vi "York DIHB - Data Processing - SNR and FFT.vi"() -> ()   [LabVIEW 2020]
doc: "Load a raw data file and calculate signal to noise ratio (SNR) & fast fourier transform (FFT). \n\nDisplays the first/largest wave in the signal."
uses:
  <vilib>/Analysis/5stat.llb/RMS (DBL).vi
  <vilib>/Utility/file.llb/Read Delimited Spreadsheet (DBL).vi
  <vilib>/measure/mascope.llb/Amplitude and Levels 1 chan.vi
  <vilib>/measure/madcrms.llb/Basic Averaged DC-RMS for 1 Chan.vi
  <vilib>/measure/maspectr.llb/FFT Spectrum (Mag-Phase) for 1 Chan.vi
  <vilib>/measure/NI_MAPro.lvlib
  <vilib>/Analysis/NI_AALPro.lvlib
panel:
  out "Signal to Noise Ratio":dbl format="%#_3g"
  out "Signal RMS Voltage":dbl format="%0.4f"
  out "Noise RMS Voltage":dbl format="%0.4f"
  out "Samples":i32
  out "Noise FFT > 250 Hz":cluster{"f0":dbl, "df":dbl, "magnitude":dbl[]}(graph)
  out "Pulse FFT":cluster{"f0":dbl, "df":dbl, "magnitude":dbl[]}(graph)
  out "Noise FFT <250 Hz":cluster{"f0":dbl, "df":dbl, "magnitude":dbl[]}(graph)
  out "Noise - Peak to Peak (V)":dbl format="%.2p"
  out "Signal - First Pulse (Volts)":waveform(dbl)(graph)
  out "Detected Frequency (Hz)":dbl format="%.2p"
  out "Noise (Volts)":waveform(dbl)(graph)
  out "Pulse Start Time (ms)":dbl
  out "DC offset (V)":dbl format="%0.2p"
  out "Peak to Peak - Amplitude (V)":dbl format="%.2p"
  out "Maximum Signal (V)":dbl format="%.2g"
  out "Minimum Signal (V)":dbl format="%.2g"
  out "Samples":i32
  out "Sampling Rate (MHz)":dbl
  out "Sampling Period (s)":dbl
  out "Raw Data - Strain Amplifier Output (Volts)":waveform(dbl)(graph)
  out "Projectile Velocity (m/s)":dbl
  out "Strain Amplifier (Volts)":dbl[](array[numeric])
  out "Time (Seconds)":dbl[](array[numeric])
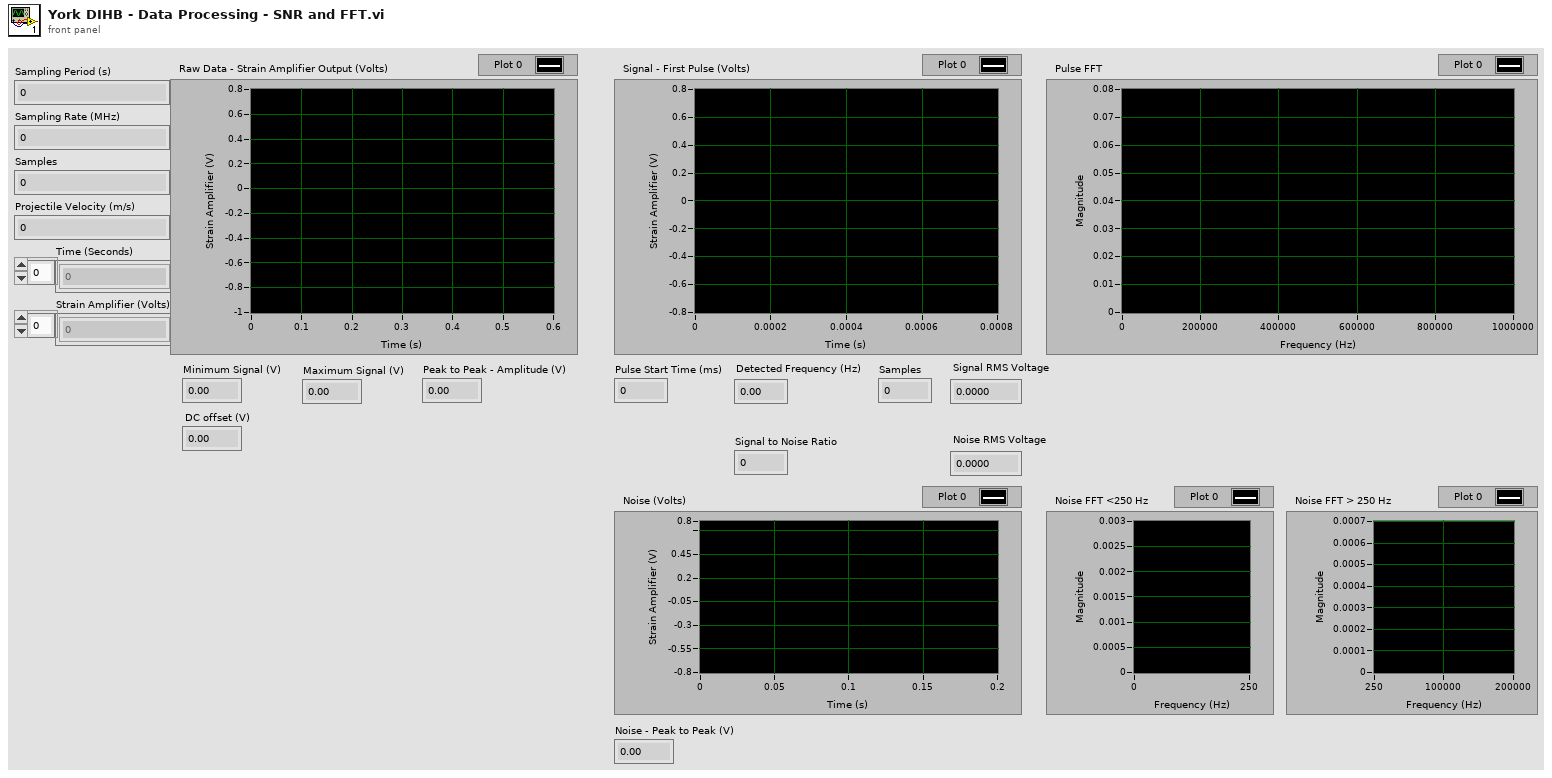
[diagram p1: front panel]
types:
  T1 = cluster{"method":enum32{"histogram", "peak", "auto select"}, "histogram size":i32, "histogram method":enum16{"mode"}, "reserved":dbl}
  T2 = typedef "LVRangeTypeDef.ctl" = cluster{"Minimum":dbl, "Maximum":dbl, "Increment":dbl, "Minor Increment":dbl, "Start":dbl}
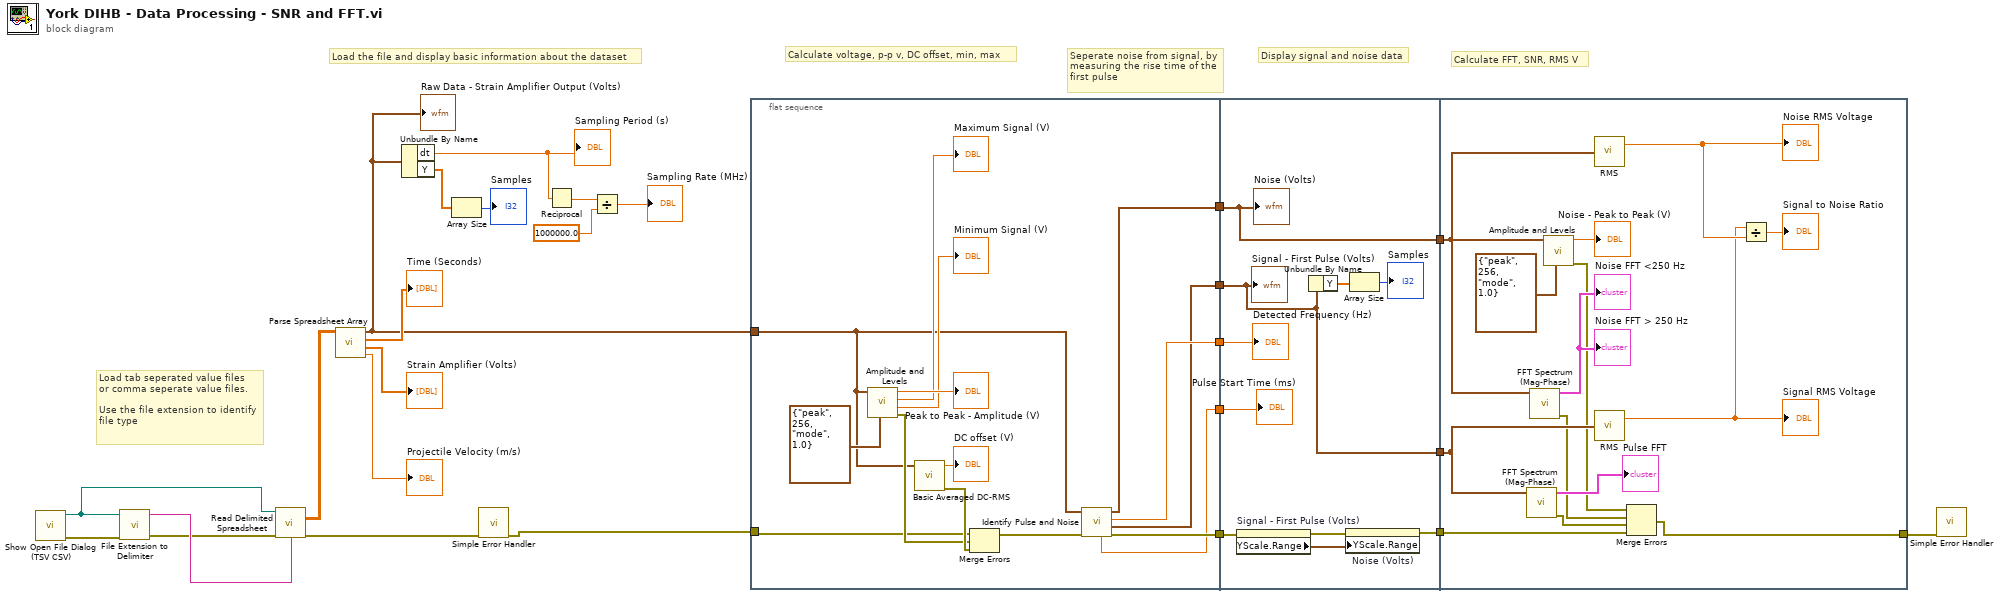
[diagram p0: block diagram]
diagram:
  # "Load tab seperated value files \nor comma seperate value files.\n\nUse the file extension to identify\nfile type"
  # "Calculate FFT, SNR, RMS V"
  # "Display signal and noise data"
  # "Seperate noise from signal, by\nmeasuring the rise time of the\nfirst pulse"
  # "Calculate voltage, p-p v, DC offset, min, max"
  # "Load the file and display basic information about the dataset"
  n1 = call "Show Open File Dialog (TSV CSV).vi"() -> ("error out"=w3:errorcluster, "selected path"=w2:path)  [unwired: 10 in]
  n2 = call "File Extension to Delimiter.vi"("error in"=w3, "Data File Path"=w2) -> ("error out"=w1:errorcluster, "Delimiter"=w7:string)  [unwired: 8 in]
  n3 = call-poly <vilib>:"Read Delimited Spreadsheet.vi"("file path (dialog if empty)"=w2, "error in (no error)"=w1, "delimiter (\\t)"=w7) -> ("all rows"=w26:dbl[][], "error out"=w6:errorcluster)  [unwired: 7 in, 4 out]
  n4 = call "Parse Spreadsheet Array.vi"("all rows"=w26) -> ("Projectile Velocity (m/s)"=→"Projectile Velocity (m/s)":dbl, "Strain Amplifier (Volts)"=→"Strain Amplifier (Volts)":dbl[], "Time (Seconds)"=→"Time (Seconds)":dbl[], "Waveform"=w8:waveform(dbl))  [unwired: 7 in]
  "Raw Data - Strain Amplifier Output (Volts)" <- w8
  n5 = Unbundle By Name(w8) -> ("dt"=w22:dbl, "Y"=w17:dbl[])
  "Sampling Period (s)" <- w22
  n6 = Array Size(array=w17) -> (size(s)=→"Samples":i32)
  n7 = call <vilib>:"Simple Error Handler.vi"("error in (no error)"=w6) -> ("error out"=w5:errorcluster)  [unwired: 4 in, 4 out]
  n8 = Reciprocal(x=w22) -> (1/x=w21:dbl)
  n9 = Divide(x=w21, y=1000000.0) -> (x/y=→"Sampling Rate (MHz)":dbl)
  n10 = flat-sequence {
    tunnel: [w32] -> w13
    tunnel: [w28] -> w12
    tunnel: [w29] -> w11
    tunnel: [w30] -> w10
    tunnel: [w27] -> w9
    tunnel: w5 -> [w34]
    tunnel: w8 -> [w31]
    tunnel: [w48] -> w16
    tunnel: [w45] -> w15
    tunnel: [w43] -> w14
    tunnel: w13 -> [w50]
    tunnel: w12 -> [w43]
    tunnel: w11 -> [w47]
    tunnel: w10 -> [w45]
    tunnel: w9 -> [w46]
    tunnel: w16 -> [w53]
    tunnel: w15 -> [w58]
    tunnel: w14 -> [w59]
    tunnel: [w52] -> w4
    frame #0 {
      n11 = call-poly <vilib>:"Amplitude and Levels.vi"("state settings"=T1 {"method"=enum."peak", "histogram size"=256, "histogram method"=enum."mode", "reserved"=1.0}, "signal in"=w31) -> ("error out"=w39:errorcluster, "low state level"=→"Minimum Signal (V)":dbl, "high state level"=→"Maximum Signal (V)":dbl, "amplitude"=→"Peak to Peak - Amplitude (V)":dbl)  [unwired: 6 in]
      n12 = call-poly <vilib>:"Basic Averaged DC-RMS.vi"("signal in"=w31) -> ("error out"=w40:errorcluster, "DC value"=→"DC offset (V)":dbl)  [unwired: 7 in, 2 out]
      n13 = Merge Errors(w34, w39, w40) -> (w41:errorcluster)
      n14 = call "Identify Pulse and Noise.vi"("error in"=w41, "Waveform In"=w31) -> ("error out"=w32:errorcluster, "Signal Waveform Out"=w28:waveform(dbl), "Detected Frequency (Hz)"=w29:dbl, "Noise Waveform Out"=w30:waveform(dbl), "Pulse Start Time (ms)"=w27:dbl)  [unwired: 5 in]
    }
    frame #1 {
      n15 = property on="Signal - First Pulse (Volts)" class="WFGraph (strict)"(error in=w50) -> (error out=w49:errorcluster, "YScale.Range"=w51:T2)  [unwired: 1 in, 1 out]
      n16 = Unbundle By Name(w43) -> ("Y"=w44:dbl[])
      n17 = property on="Noise (Volts)" class="WFGraph (strict)"(error in=w49, "YScale.Range"=w51) -> (error out=w48:errorcluster)  [unwired: 1 in, 1 out]
      n18 = Array Size(array=w44) -> (size(s)=→"Samples":i32)
      "Pulse Start Time (ms)" <- w46
      "Noise (Volts)" <- w45
      "Detected Frequency (Hz)" <- w47
      "Signal - First Pulse (Volts)" <- w43
    }
    frame #2 {
      n19 = call-poly <vilib>:"FFT Spectrum (Mag-Phase).vi"("time signal"=w59) -> ("error out"=w54:errorcluster, "magnitude"=→"Pulse FFT":cluster{"f0":dbl, "df":dbl, "magnitude":dbl[]})  [unwired: 6 in, 3 out]
      n20 = call-poly <vilib>:"FFT Spectrum (Mag-Phase).vi"("time signal"=w58) -> ("error out"=w55:errorcluster, "magnitude"=→"Noise FFT <250 Hz" →"Noise FFT > 250 Hz":cluster{"f0":dbl, "df":dbl, "magnitude":dbl[]})  [unwired: 6 in, 3 out]
      n21 = call-poly <vilib>:"Amplitude and Levels.vi"("state settings"=T1 {"method"=enum."peak", "histogram size"=256, "histogram method"=enum."mode", "reserved"=1.0}, "signal in"=w58) -> ("error out"=w56:errorcluster, "amplitude"=→"Noise - Peak to Peak (V)":dbl)  [unwired: 6 in, 2 out]
      n22 = call-poly <vilib>:"RMS.vi"("X"=w58) -> ("rms value"=w64:dbl)  [unwired: 1 out]
      "Noise RMS Voltage" <- w64
      n23 = call-poly <vilib>:"RMS.vi"("X"=w59) -> ("rms value"=w63:dbl)  [unwired: 1 out]
      "Signal RMS Voltage" <- w63
      n24 = Merge Errors(w56, w55, w54, w53) -> (w52:errorcluster)
      n25 = Divide(x=w63, y=w64) -> (x/y=→"Signal to Noise Ratio":dbl)
    }
  }
  n26 = call <vilib>:"Simple Error Handler.vi"("error in (no error)"=w4) -> ()  [unwired: 4 in, 5 out]
